vi "Updateinter.vi"(10 "更新包远端地址":string="/updatefiles/OneStation/V4/一体化微型水质监测站.zip", 11 "测试版？":bool) -> ()   [LabVIEW 2016, in "数据传输系统-05.lvlib" / "update.lvlib"]
uses:
  update.lvlib
  <vilib>/Utility/miscctls.llb/LVPointTypeDef.ctl
  http client class/http client.lvclass
panel:
  out "已下载大小":sgl format="%.2f MB"
  out "滑动杆":dbl(slide) scale=0.0..100.0
  in  "取消按钮":bool
  out "last status string":string caption="最近状态字符串"
  out "command":string caption="命令"
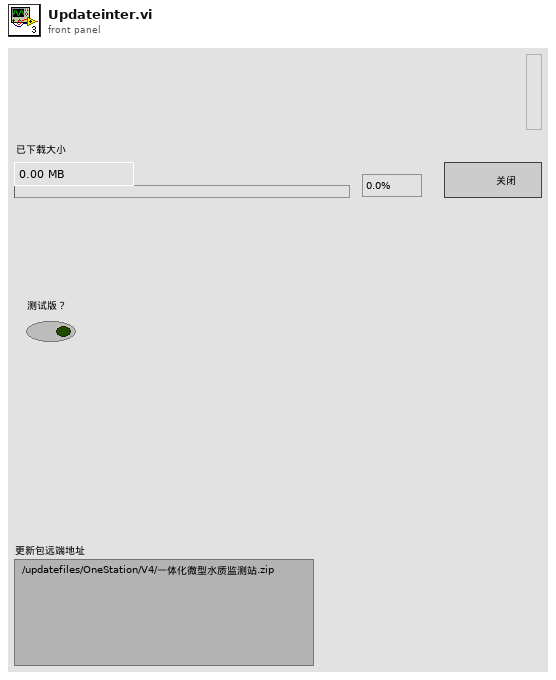
[diagram p1: front panel]
types:
  T1 = typedef "LVPointTypeDef.ctl" = cluster{"Horizontal":i16, "Vertical":i16}
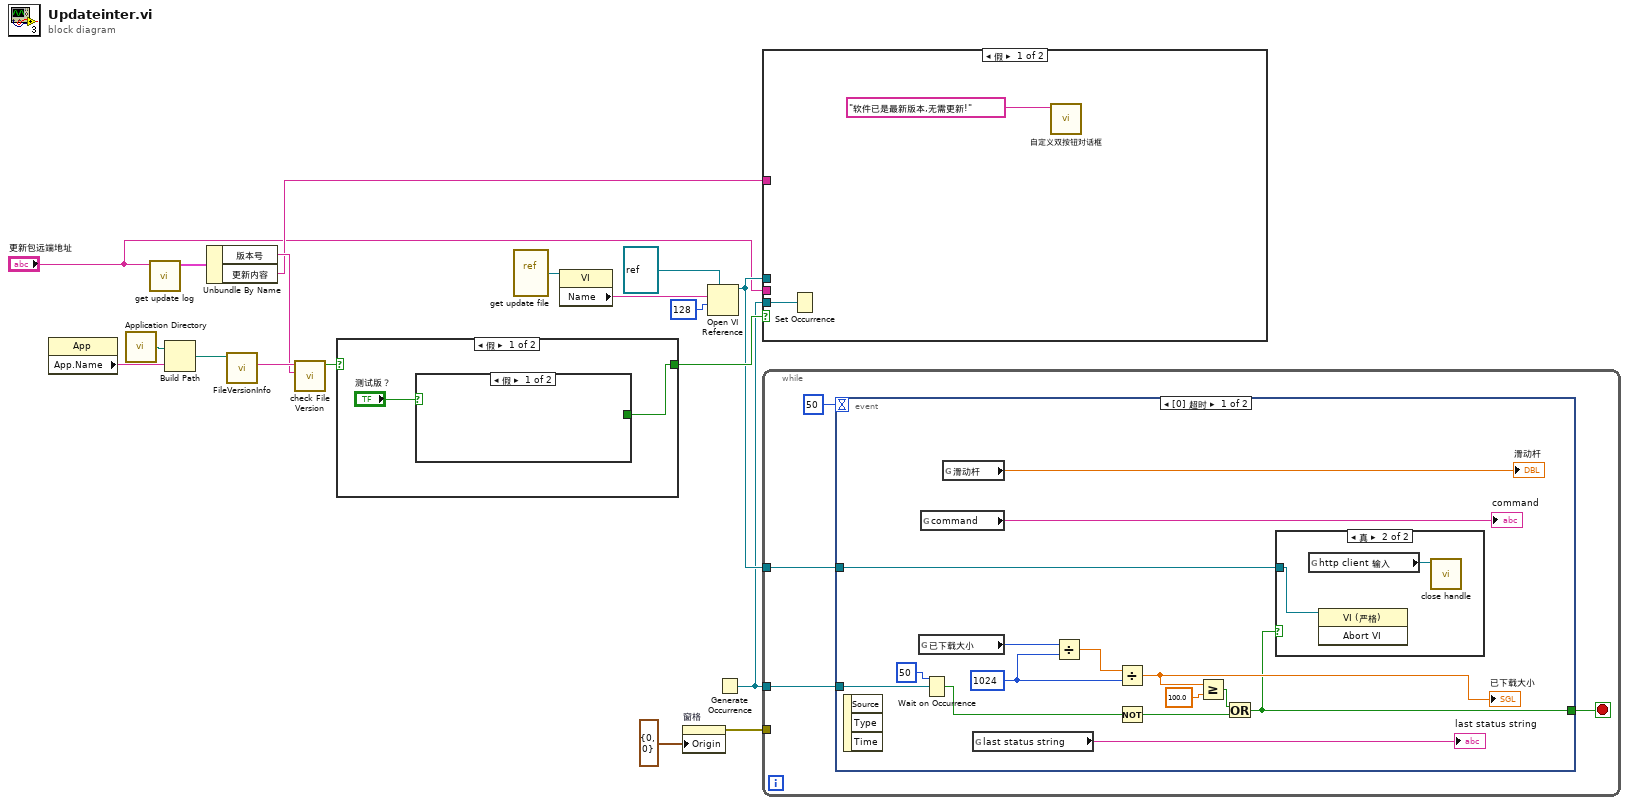
[diagram p0: block diagram]
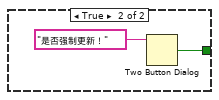
[diagram p2: hidden frame]
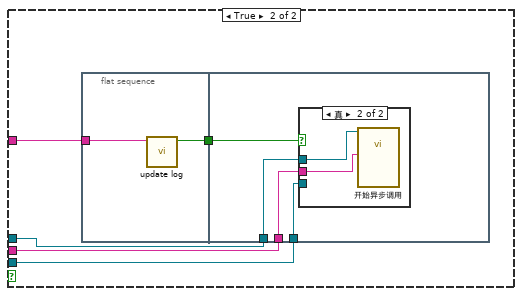
[diagram p4: hidden frame]
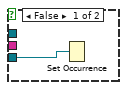
[diagram p5: hidden frame]
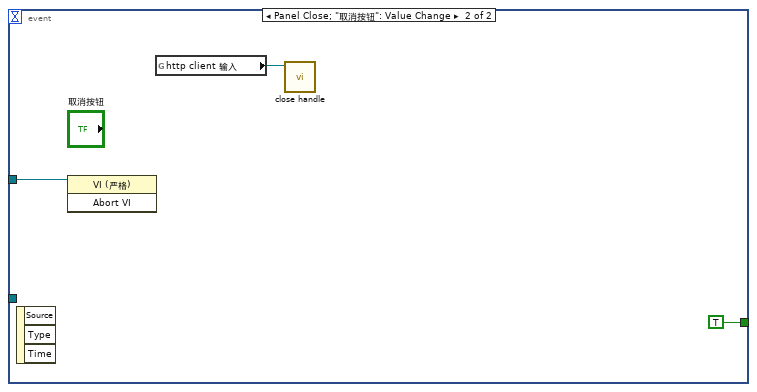
[diagram p7: hidden frame]
diagram:
  n1 = property class="App"() -> ("App.Name"=w18:string)  [unwired: 2 in, 2 out]
  n2 = call <vilib>:"Application Directory.vi"() -> ("Application Directory"=w10:path)
  n3 = call "get update log.vi"("远端地址"="更新包远端地址") -> ("元素"=w11:cluster{"版本号":string, "更新内容":string})  [unwired: 8 in, 2 out]
  n4 = Build Path(base path=w10, name or relative path=w18) -> (appended path=w17:path)
  n5 = Unbundle By Name(w11) -> ("版本号"=w9:string, "更新内容"=w8:string)
  n6 = call <vilib>:"FileVersionInfo.vi"("Application Path in"=w17) -> ("File Version Info"=w16:string)  [unwired: 7 in, 3 out]
  n7 = call "check File Version.vi"("remote File Version Info"=w9, "Local File Version Info"=w16) -> ("new?"=w15:bool)  [unwired: 9 in]
  n8 = case shown="假" w15 {
    selector: w15 -> [_ w23]
    tunnel: [w19 w23] -> w14
    frame False {
      n9 = case shown="假" "测试版？" {
        tunnel: [_ w22] -> w19
        frame False {
        }
        frame True {
          n10 = Two Button Dialog(message="是否强制更新！" ("消息")) -> (T button?=w22:bool)  [unwired: 2 in]
        }
      }
    }
    frame True {
    }
  }
  n11 = vi-ref "get update file.vi"() -> (w4:refnum<vi>)
  n12 = property class="VI"(reference=w4) -> ("Name"=w5:string)  [unwired: 1 in, 2 out]
  n13 = property on="窗格" class="Pane"("Origin"=T1 {"Horizontal"=0, "Vertical"=0} ("原点")) -> (error out=w13:errorcluster)  [unwired: 2 in, 1 out]
  n14 = Open VI Reference(type specifier VI Refnum (for type only)=refnum<vi> refnum, vi path=w5, options=128 ("选项")) -> (vi reference=w3:refnum<vi>)  [unwired: 3 in, 1 out]
  n15 = Generate Occurrence() -> (w2:refnum<k4>)
  n16 = case shown="假" w14 {
    tunnel: w8 -> [_ w30]
    tunnel: "更新包远端地址" -> [_ w28]
    tunnel: w3 -> [_ w27]
    tunnel: w2 -> [w24 w26]
    frame False {
      n17 = Set Occurrence(w24) -> ()
      n18 = call "自定义双按钮对话框.vi"("消息"="软件已是最新版本,无需更新!") -> ()  [unwired: 10 in, 1 out]
    }
    frame True {
      n19 = flat-sequence {
        tunnel: w30 -> [w32]
        tunnel: [w31] -> w29
        tunnel: w29 -> [w36]
        tunnel: w28 -> [w35]
        tunnel: w27 -> [w34]
        tunnel: w26 -> [w33]
        frame #0 {
          n20 = call "update log.vi"("更新记录"=w32) -> ("check"=w31:bool)  [unwired: 10 in]
        }
        frame #1 {
          n21 = case shown="真" w36 {
            tunnel: w35 -> [_ w39]
            tunnel: w34 -> [_ w38]
            tunnel: w33 -> [w37 _]
            frame False {
              n22 = Set Occurrence(w37) -> ()
            }
            frame True {
              n23 = call-by-ref "开始异步调用"(reference=w38, "远端地址"=w39) -> ()  [unwired: 11 in, 3 out]
            }
          }
        }
      }
    }
  }
  n24 = while {
    tunnel: w13 -> [_]
    tunnel: w3 -> [w41]
    tunnel: w2 -> [w40]
    stop <- w42 stop-if-true
    n25 = event shown="[0] 超时" {
      selector: _ -> [_ _]
      dyn-events: _ -> [_ _]
      timeout: 50 -> [_ _]
      tunnel: [w44 TRUE] -> w42
      tunnel: w41 -> [w45 w62]
      tunnel: w40 -> [w52 _]
      event Timeout {
        w53 = i64 1024 ("y")
        n26 = event-data() -> ()  [unwired: 1 in, 3 out]
        n27 = global read "更新全局变量.vi" "已下载大小"() -> (w55:i64)
        n28 = global read "更新全局变量.vi" "command"() -> (→"command":string)
        n29 = Wait on Occurrence(2:w52, 3:50 ("毫秒超时(-1)")) -> (0:w50:bool)  [unwired: 1 in]
        n30 = global read "更新全局变量.vi" "滑动杆"() -> (→"滑动杆":dbl)
        n31 = global read "更新全局变量.vi" "last status string"() -> (→"last status string":string)
        n32 = Divide(x=w55, y=w53) -> (x/y=w54:dbl)
        n33 = Divide(x=w54, y=w53) -> (x/y=w48:dbl)
        "已下载大小" <- w48
        n34 = Not(x=w50) -> (.not. x?=w49:bool)
        n35 = Greater Or Equal?(x=w48, y=100.0) -> (x >= y?=w46:bool)
        n36 = Or(x=w46, y=w49) -> (x .or. y?=w44:bool)
        n37 = case shown="真" w44 {
          tunnel: w45 -> [_ w59]
          frame False {
          }
          frame True {
            n38 = global read "更新全局变量.vi" "http client 输入"() -> (w60:refnum<class "http client.lvclass">)
            n39 = invoke class="VI (严格)" method="Abort VI"(reference=w59) -> ()  [unwired: 2 in, 3 out]
            n40 = call "close handle.vi"("http client 输入"=w60) -> ()  [unwired: 9 in, 2 out]
          }
        }
      }
      event Panel Close; "取消按钮": Value Change {
        n41 = event-data() -> ()  [unwired: 1 in, 3 out]
        n42 = invoke class="VI (严格)" method="Abort VI"(reference=w62) -> ()  [unwired: 2 in, 3 out]
        n43 = global read "更新全局变量.vi" "http client 输入"() -> (w61:refnum<class "http client.lvclass">)
        n44 = call "close handle.vi"("http client 输入"=w61) -> ()  [unwired: 9 in, 2 out]
      }
    }
  }
